vi "Net Weight.vi"(8 "error in (no error)":errorcluster, 11 "Instrument.LN2 in":refnum<class "Instrument.LN2.lvclass">) -> (0 "error out":errorcluster, 2 "Net Weight (kg)":dbl, 3 "Instrument.LN2 out":refnum<class "Instrument.LN2.lvclass">)   [LabVIEW 2019, in "Instrument.LN2.lvclass"]
uses:
  Instrument.LN2.lvclass
  Instrument.LN2.lvclass/Instrument.LN2.ctl
  <vilib>/regexp/Match Regular Expression.xnode
panel:
  out "before match":string
  out "after match":string
  out "return count":u32
  out "VISA resource name out":refnum<visa-resource-name>
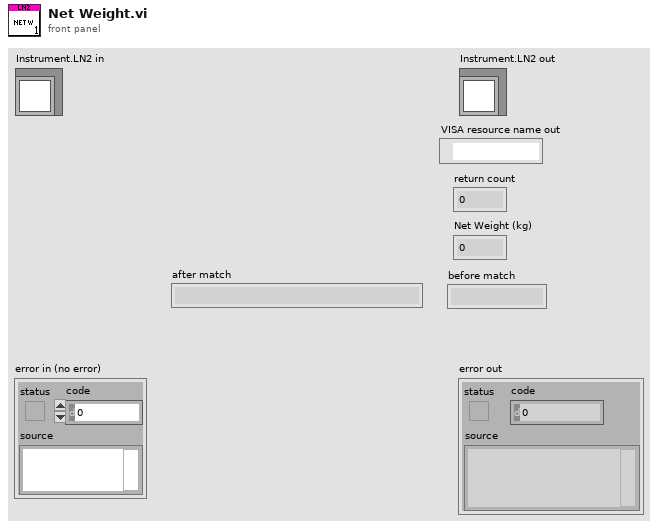
[diagram p1: front panel]
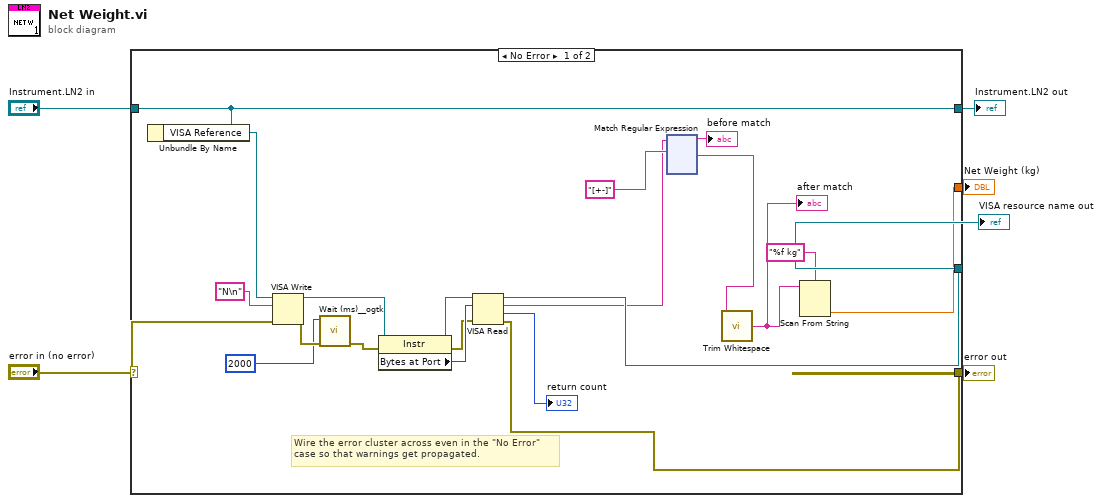
[diagram p0: block diagram]
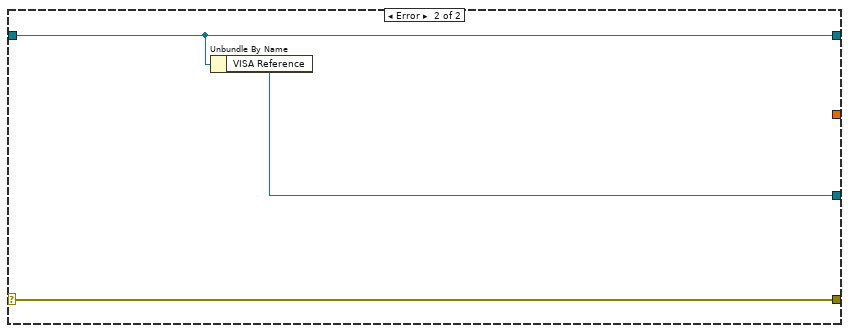
[diagram p2: hidden frame]
diagram:
  n1 = case shown="No Error" "error in (no error)" {
    selector: "error in (no error)" -> [w23 w144]
    tunnel: [w25 w144] -> w5
    tunnel: [w27 w143] -> w3
    tunnel: "Instrument.LN2 in" -> [w27 w143]
    tunnel: [w24 w142] -> w2
    tunnel: [w7 _] -> w1
    frame No Error {
      # "Wire the error cluster across even in the \"No Error\"\ncase so that warnings get propagated."
      n2 = Unbundle By Name(w27) -> ("VISA Reference"=w26:refnum<visa-resource-name>)
      n3 = VISA Write(VISA resource name=w26, write buffer="N\n", error in (no error)=w23) -> (VISA resource name out=w19:refnum<visa-resource-name>, error out=w17:errorcluster)  [unwired: 1 out]
      n4 = call <userlib>:"Wait (ms)__ogtk.vi"("error in (no error)"=w17, "milliseconds to wait"=u32 2000) -> ("error out"=w16:errorcluster)  [unwired: 8 in, 1 out]
      n5 = property class="Instr"(reference=w19, error in=w16) -> (reference out=w18:refnum<visa-resource-name>, error out=w15:errorcluster, "Bytes at Port"=w20:u32)
      n6 = VISA Read(VISA resource name=w18, byte count=w20, error in (no error)=w15) -> (VISA resource name out=w24:refnum<visa-resource-name>, read buffer=w8:string, return count=→"return count":u32, error out=w25:errorcluster)
      n7 = xnode "Match Regular Expression"("input string"=w8, "regular expression"="[+-]" ("format string")) -> ("before match"=→"before match":string, "after match"=w10:string)  [unwired: 4 in, 3 out]
      n8 = call <vilib>:"Trim Whitespace.vi"("string"=w10) -> ("trimmed string"=w9:string)  [unwired: 1 in]
      "after match" <- w9
      n9 = Scan From String(format string="%f kg", input string=w9) -> (output 1=w7:dbl)  [unwired: 3 in, 3 out]
    }
    frame Error {
      n10 = Unbundle By Name(w143) -> ("VISA Reference"=w142:refnum<visa-resource-name>)
    }
  }
  "error out" <- w5
  "Instrument.LN2 out" <- w3
  "Net Weight (kg)" <- w1
  "VISA resource name out" <- w2
